vi "Tx.vi"(8 "error in (no error)":errorcluster, 10 "Command Parameters":T1, 11 "Dispatcher in":refnum<class "Dispatcher.lvclass">) -> (0 "error out":errorcluster, 3 "Dispatcher out":refnum<class "Dispatcher.lvclass">)   [LabVIEW 2017, in "DSF Core.lvlib" / "Dispatcher.lvclass"]
uses:
  Dispatcher.lvclass
  Interfaces/Dispatcher/Parameters.ctl
  Interfaces/Dispatcher/Tx Parameters.ctl
  Interfaces/Transceiver Interface/Command.ctl
  Dispatcher.lvclass/Dispatcher.ctl
  Plugin/Plugin.lvclass/Plugin.ctl
  Plugin/Plugin.lvclass
  Interfaces/Transceiver Interface/Plugin Interface.lvclass
  Interfaces/Dispatcher/Dispatcher Interface.lvclass
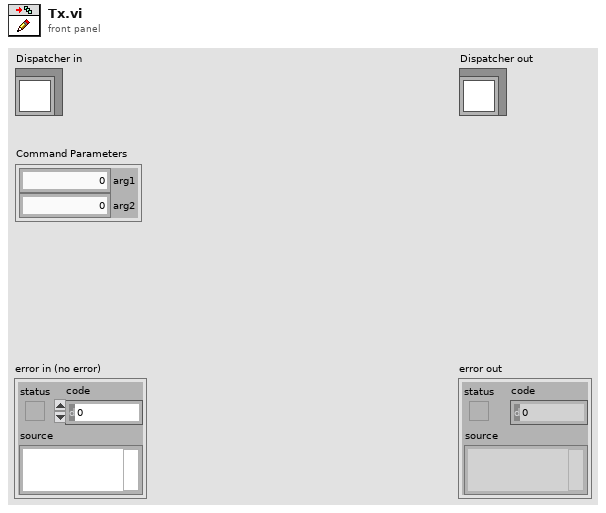
[diagram p1: front panel]
types:
  T1 = typedef "DSF Core.lvlib/Dispatcher Interface.lvclass/Parameters.ctl" = cluster{"arg1":u64, "arg2":u64}
  T2 = typedef "DSF Core.lvlib/Plugin Interface.lvclass/Command.ctl" = enum8{"Set Base Pointer", "Rx", "Tx", "Shutdown"}
  T3 = typedef "DSF Core.lvlib/Dispatcher Interface.lvclass/Tx Parameters.ctl" = cluster{"Plugin ID":i32, "Transfer Group ID":i32, "Iteration":u64}
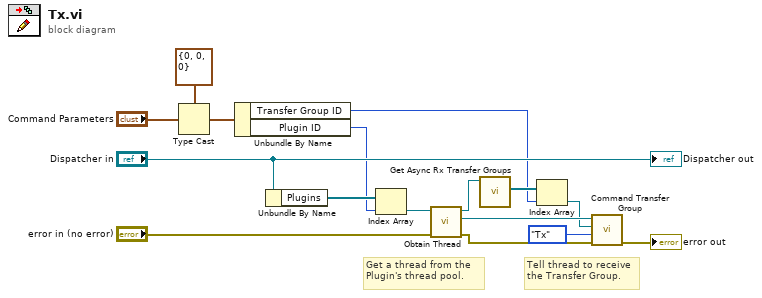
[diagram p0: block diagram]
diagram:
  # "Tell thread to receive the Transfer Group."
  # "Get a thread from the Plugin's thread pool."
  n1 = Type Cast(type=T3 {"Plugin ID"=0, "Transfer Group ID"=0, "Iteration"=0}, x="Command Parameters") -> (*(type *) &x=w14:T3)
  n2 = Unbundle By Name(w14) -> ("Transfer Group ID"=w9:i32, "Plugin ID"=w10:i32)
  n3 = Unbundle By Name("Dispatcher in") -> ("Plugins"=w13:refnum<class "Plugin.lvclass">[])
  n4 = Index Array(array=w13, index=w10) -> (element=w7:refnum<class "Plugin.lvclass">)
  n5 = call "Obtain Thread.vi"("error in (no error)"="error in (no error)", "Plugin in"=w7) -> ("error out"=w3:errorcluster, "Plugin Thread Interface"=w8:refnum<class "Plugin Interface.lvclass">, "Plugin out"=w6:refnum<class "Plugin.lvclass">)  [unwired: 7 in]
  n6 = call "Get Async Rx Transfer Groups.vi"("Plugin in"=w6) -> ("Async Rx Transfer Groups"=w11:refnum<class "Transfer Group.lvclass">[])  [unwired: 9 in, 1 out]
  n7 = Index Array(array=w11, index=w9) -> (element=w5:refnum<class "Transfer Group.lvclass">)
  n8 = call "Command Transfer Group.vi"("error in (no error)"=w3, "Command"=Command."Tx", "Transfer Group"=w5, "Plugin Interface in"=w8) -> ("error out"=→"error out":errorcluster)  [unwired: 6 in, 1 out]
  "Dispatcher out" <- "Dispatcher in"
